vi "ParseBounceData.vi"(5 "Data_In":string="b'OK\\n\\r'\r\nDMA Length: 43008\r\nTx_1 Rx_1: {'Frequency': 'Passed', 'Power': 'Passed'}\r\nMax Value: -5.066 dBFS at -6.226 MHz\r\nTx_2 Rx_1: {'Frequency': 'Passed', 'Power': 'Passed'}\r\nMax Value: -6.924 dBFS at -6.226 MHz\r\nTx_1 Rx_2: {'Frequency': 'Passed', 'Power': 'Passed'}\r\nMax Value: -6.565 dBFS at -6.152 MHz\r\nTx_3 Rx_1: {'Frequency': 'Passed', 'Power': 'Passed'}\r\nMax Value: -6.967 dBFS at -6.226 MHz\r\nTx_2 Rx_2: {'Frequency': 'Passed', 'Power': 'Passed'}\r\nMax Value: -6.388 dBFS at -6.226 MHz\r\nTx_4 Rx_1: {'Frequency': 'Passed', 'Power': 'Passed'}\r\nMax Value: -6.945 dBFS at -6.226 MHz\r\nTx_3 Rx_2: {'Frequency': 'Passed', 'Power': 'Passed'}\r\nMax Value: -6.080 dBFS at -6.152 MHz\r\nTx_2 Rx_3: {'Frequency': 'Passed', 'Power': 'Passed'}\r\nMax Value: -5.226 dBFS at -6.152 MHz\r\nTx_4 Rx_2: {'Frequency': 'Passed', 'Power': 'Passed'}\r\nMax Value: -6.517 dBFS at -6.226 MHz\r\nTx_3 Rx_3: {'Frequency': 'Passed', 'Power': 'Passed'}\r\nMax Value: -5.453 dBFS at -6.226 MHz\r\nTx_5 Rx_2: {'Frequency': 'Passed', 'Power': 'Passed'}\r\nMax Value: -6.717 dBFS at -6.226 MHz\r\nTx_4 Rx_3: {'Frequency': 'Passed', 'Power': 'Passed'}\r\nMax Value: -5.646 dBFS at -6.226 MHz\r\nTx_3 Rx_4: {'Frequency': 'Passed', 'Power': 'Passed'}\r\nMax Value: -5.349 dBFS at -6.152 MHz\r\nTx_5 Rx_3: {'Frequency': 'Passed', 'Power': 'Passed'}\r\nMax Value: -5.643 dBFS at -6.226 MHz\r\nTx_4 Rx_4: {'Frequency': 'Passed', 'Power': 'Passed'}\r\nMax Value: -5.707 dBFS at -6.226 MHz\r\nTx_6 Rx_3: {'Frequency': 'Passed', 'Power': 'Passed'}\r\nMax Value: -5.844 dBFS at -6.226 MHz\r\nTx_5 Rx_4: {'Frequency': 'Passed', 'Power': 'Passed'}\r\nMax Value: -5.505 dBFS at -6.226 MHz\r\nTx_7 Rx_3: {'Frequency': 'Passed', 'Power': 'Passed'}\r\nMax Value: -5.223 dBFS at -6.152 MHz\r\nTx_6 Rx_4: {'Frequency': 'Passed', 'Power': 'Passed'}\r\nMax Value: -5.202 dBFS at -6.226 MHz\r\nTx_5 Rx_5: {'Frequency': 'Passed', 'Power': 'Passed'}\r\nMax Value: -5.983 dBFS at -6.226 MHz\r\nTx_7 Rx_4: {'Frequency': 'Passed', 'Power': 'Passed'}\r\nMax Value: -5.318 dBFS at -6.226 MHz\r\nTx_6 Rx_5: {'Frequency': 'Passed', 'Power': 'Passed'}\r\nMax Value: -5.734 dBFS at -6.226 MHz\r\nTx_8 Rx_4: {'Frequency': 'Passed', 'Power': 'Passed'}\r\nMax Value: -5.205 dBFS at -6.226 MHz\r\nTx_7 Rx_5: {'Frequency': 'Passed', 'Power': 'Passed'}\r\nMax Value: -5.248 dBFS at -6.226 MHz\r\nTx_6 Rx_6: {'Frequency': 'Passed', 'Power': 'Passed'}\r\nMax Value: -5.428 dBFS at -6.226 MHz\r\nTx_8 Rx_5: {'Frequency': 'Passed', 'Power': 'Passed'}\r\nMax Value: -5.738 dBFS at -6.226 MHz\r\nTx_7 Rx_6: {'Frequency': 'Passed', 'Power': 'Passed'}\r\nMax Value: -5.289 dBFS at -6.226 MHz\r\nTx_9 Rx_5: {'Frequency': 'Passed', 'Power': 'Passed'}\r\nMax Value: -6.211 dBFS at -6.226 MHz\r\nTx_8 Rx_6: {'Frequency': 'Passed', 'Power': 'Passed'}\r\nMax Value: -5.201 dBFS at -6.226 MHz\r\nTx_10 Rx_5: {'Frequency': 'Passed', 'Power': 'Passed'}\r\nMax Value: -6.328 dBFS at -6.226 MHz\r\nTx_9 Rx_6: {'Frequency': 'Passed', 'Power': 'Passed'}\r\nMax Value: -6.355 dBFS at -6.226 MHz\r\nTx_8 Rx_7: {'Frequency': 'Passed', 'Power': 'Passed'}\r\nMax Value: -5.296 dBFS at -6.226 MHz\r\nTx_10 Rx_6: {'Frequency': 'Passed', 'Power': 'Passed'}\r\nMax Value: -6.349 dBFS at -6.226 MHz\r\nTx_9 Rx_7: {'Frequency': 'Passed', 'Power': 'Passed'}\r\nMax Value: -6.183 dBFS at -6.226 MHz\r\nTx_11 Rx_6: {'Frequency': 'Passed', 'Power': 'Passed'}\r\nMax Value: -6.896 dBFS at -6.226 MHz\r\nTx_10 Rx_7: {'Frequency': 'Passed', 'Power': 'Passed'}\r\nMax Value: -6.724 dBFS at -6.226 MHz\r\nTx_9 Rx_8: {'Frequency': 'Passed', 'Power': 'Passed'}\r\nMax Value: -6.414 dBFS at -6.226 MHz\r\nTx_11 Rx_7: {'Frequency': 'Passed', 'Power': 'Passed'}\r\nMax Value: -6.283 dBFS at -6.226 MHz\r\nTx_10 Rx_8: {'Frequency': 'Passed', 'Power': 'Passed'}\r\nMax Value: -6.328 dBFS at -6.226 MHz\r\nTx_12 Rx_7: {'Frequency': 'Passed', 'Power': 'Passed'}\r\nMax Value: -5.939 dBFS at -6.226 MHz\r\nTx_11 Rx_8: {'Frequency': 'Passed', 'Power': 'Passed'}\r\nMax Value: -6.370 dBFS at -6.226 MHz\r\nTx_12 Rx_8: {'Frequency': 'Passed', 'Power': 'Passed'}\r\nMax Value: -6.672 dBFS at -6.226 MHz\r\n", 11 "error in":errorcluster) -> (2 "P/F_power":bool, 3 "Passed?(T)":bool, 6 "Data_Out":string[][](array[string]), 15 "error out":errorcluster)   [LabVIEW 2018]
panel:
  out "P/F_freq":bool[](array[boolean])
  out "Array 3":string[](array[string])
  out "Array 2":string[](array[string])
  out "mhz":string[](array[string])
  out "dbfs":string[](array[string])
  out "rx":string[](array[string])
  out "tx":string[](array[string])
  out "Formatted_ary":string[][](array[string])
  out "size_match?(t)":bool
  out "Data_index":i32[](array[numeric])
  out "Tx_index":i32[](array[numeric])
  out "spreadsheet string":string
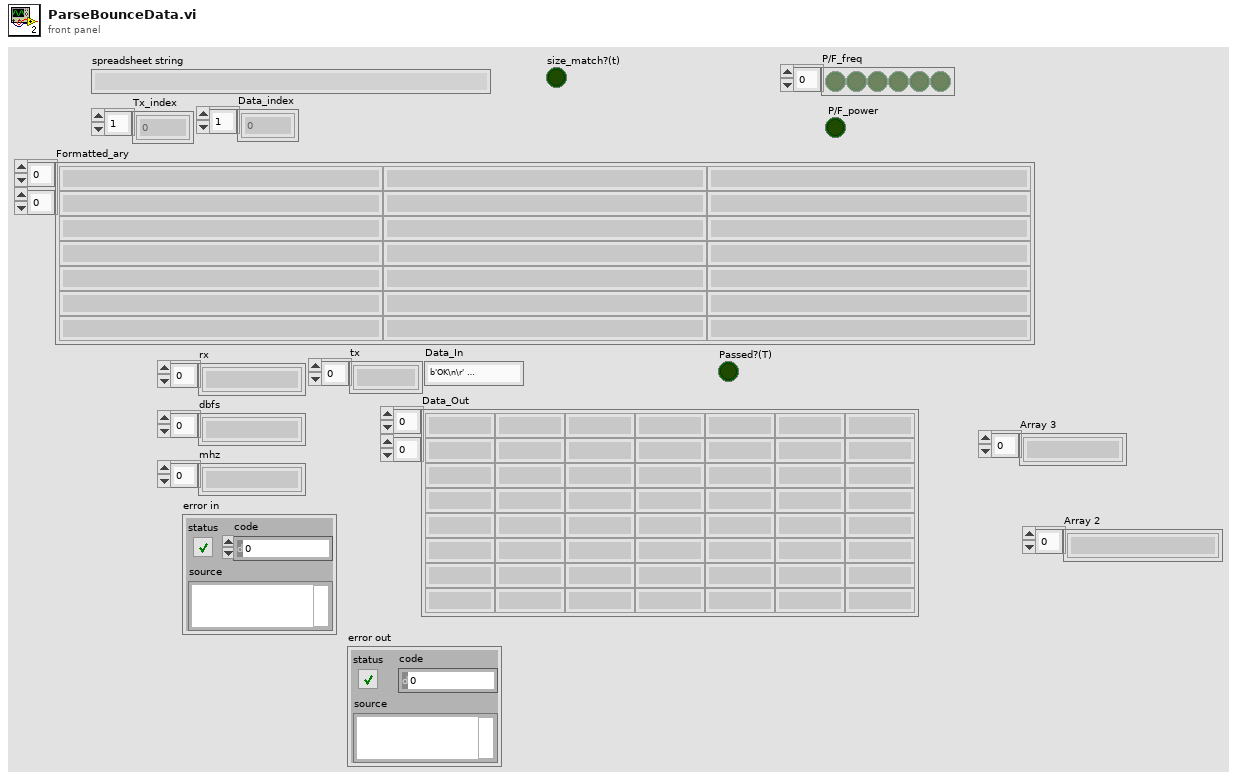
[diagram p1: front panel]
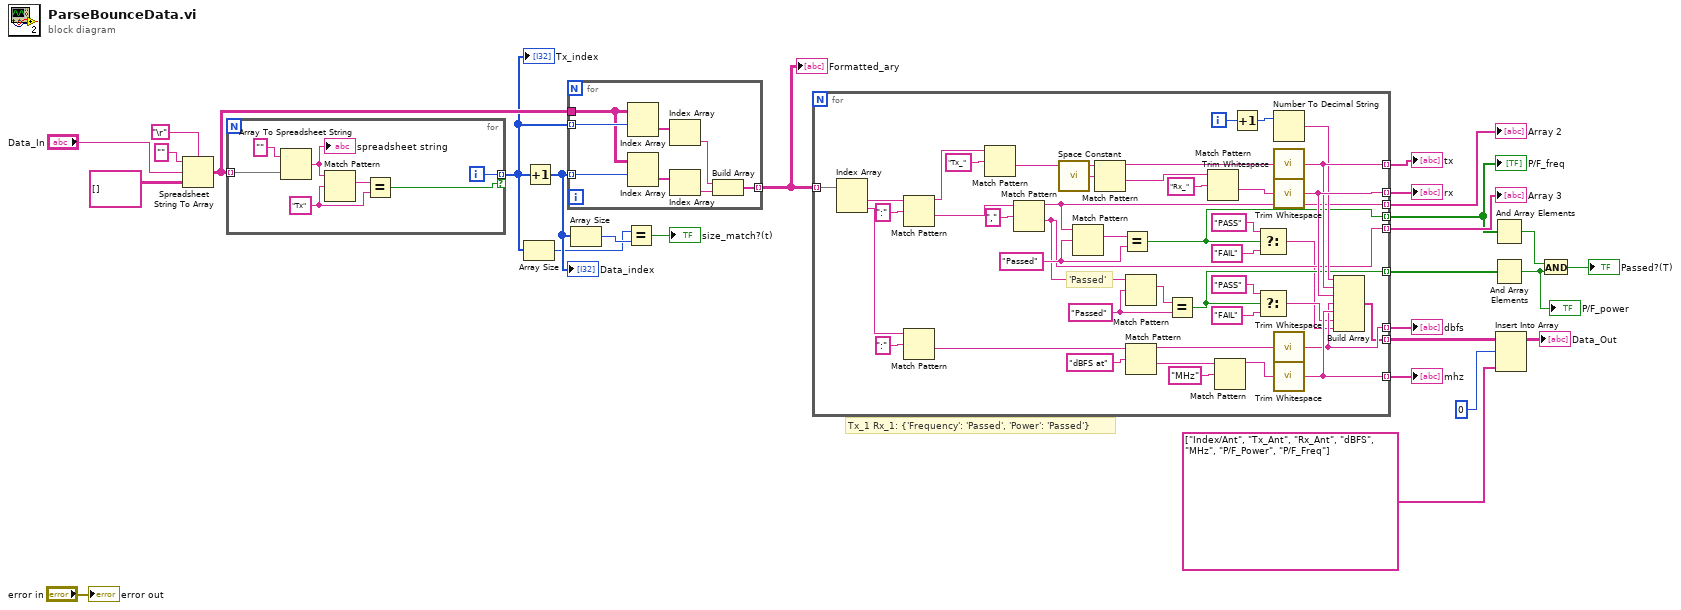
[diagram p0: block diagram]
diagram:
  # "Tx_1 Rx_1: {'Frequency': 'Passed', 'Power': 'Passed'}"
  n1 = Spreadsheet String To Array(delimiter (Tab)="\r", format string="", spreadsheet string="Data_In", array type (2D Dbl)=string[][] []) -> (array=w23:string[][])
  n2 = for {
    tunnel: w23 -> [w34] mode=indexing
    tunnel: [w29] -> w21 mode=indexing if=w28
    i -> [w29]
    w30 = "Tx" ("regular expression")
    n3 = Array To Spreadsheet String(array=w34, 3:"" ("format string")) -> (spreadsheet string=w32:string)  [unwired: 1 in]
    "spreadsheet string" <- w32
    n4 = Match Pattern(string=w32, regular expression=w30) -> (match substring=w31:string)  [unwired: 1 in, 3 out]
    n5 = Equal?(x=w31, y=w30) -> (x = y?=w28:bool)
  }
  "Tx_index" <- w21
  n6 = Array Size(array=w21) -> (size(s)=w19:i32)
  n7 = Increment(x=w21) -> (x+1=w22:i32[])
  "Data_index" <- w22
  n8 = for {
    tunnel: w23 -> [w39]
    tunnel: w22 -> [w42] mode=indexing
    tunnel: w21 -> [w40] mode=indexing
    tunnel: [w35] -> w17 mode=indexing
    n9 = Index Array(array=w39, index (row)=w40) -> (element=w38:string[])  [unwired: 1 in]
    n10 = Index Array(array=w39, index (row)=w42) -> (element=w41:string[])  [unwired: 1 in]
    n11 = Index Array(array=w38) -> (element=w37:string)  [unwired: 1 in]
    n12 = Index Array(array=w41) -> (element=w36:string)  [unwired: 1 in]
    n13 = Build Array(w37, w36) -> (w35:string[])
  }
  "Formatted_ary" <- w17
  n14 = Array Size(array=w22) -> (size(s)=w20:i32)
  n15 = Equal?(x=w19, y=w20) -> (x = y?=→"size_match?(t)":bool)
  n16 = for {
    tunnel: w17 -> [w85] mode=indexing
    tunnel: [w63] -> w16 mode=indexing
    tunnel: [w64] -> w15 mode=indexing
    tunnel: [w65] -> w14 mode=indexing
    tunnel: [w66] -> w13 mode=indexing
    tunnel: [w62] -> w12 mode=indexing
    tunnel: [w56] -> w8 mode=indexing
    tunnel: [w51] -> w7 mode=indexing
    tunnel: [w50] -> w6 mode=indexing
    tunnel: [w45] -> w5 mode=indexing
    i -> [w60]
    w53 = "Passed"
    w54 = "Passed"
    # "'Passed'"
    n17 = Index Array(array=w85) -> (element #1=w77:string, element #2=w73:string)  [unwired: 2 in]
    n18 = Match Pattern(string=w77, regular expression=":") -> (before substring=w81:string, after substring=w58:string)  [unwired: 1 in, 2 out]
    n19 = Match Pattern(string=w73, regular expression=":") -> (after substring=w72:string)  [unwired: 1 in, 3 out]
    n20 = Match Pattern(string=w81, regular expression="Tx_") -> (after substring=w80:string)  [unwired: 1 in, 3 out]
    n21 = Match Pattern(string=w58, regular expression=",") -> (before substring=w56:string, after substring=w51:string)  [unwired: 1 in, 2 out]
    n22 = call <vilib>:"Space Constant.vi"() -> ("String"=w79:string)
    n23 = Match Pattern(string=w56, regular expression=w54) -> (match substring=w55:string)  [unwired: 1 in, 3 out]
    n24 = Match Pattern(string=w80, regular expression=w79) -> (before substring=w78:string, after substring=w76:string)  [unwired: 1 in, 2 out]
    n25 = Equal?(x=w55, y=w54) -> (x = y?=w50:bool)
    n26 = Match Pattern(string=w51, regular expression=w53) -> (match substring=w52:string)  [unwired: 1 in, 3 out]
    n27 = Match Pattern(string=w72, regular expression="dBFS at") -> (before substring=w70:string, after substring=w69:string)  [unwired: 1 in, 2 out]
    n28 = Equal?(x=w52, y=w53) -> (x = y?=w45:bool)
    n29 = Match Pattern(string=w76, regular expression="Rx_") -> (after substring=w75:string)  [unwired: 1 in, 3 out]
    n30 = Match Pattern(string=w69, regular expression="MHz") -> (before substring=w67:string)  [unwired: 1 in, 3 out]
    n31 = Increment(x=w60) -> (x+1=w59:i32)
    n32 = Select(t="PASS", s=w50, f="FAIL") -> (s? t:f=w43:string)
    n33 = Select(t="PASS", s=w45, f="FAIL") -> (s? t:f=w44:string)
    n34 = Number To Decimal String(number=w59) -> (decimal integer string=w61:string)  [unwired: 1 in]
    n35 = call <vilib>:"Trim Whitespace.vi"("string"=w78) -> ("trimmed string"=w63:string)  [unwired: 1 in]
    n36 = call <vilib>:"Trim Whitespace.vi"("string"=w75) -> ("trimmed string"=w64:string)  [unwired: 1 in]
    n37 = call <vilib>:"Trim Whitespace.vi"("string"=w70) -> ("trimmed string"=w65:string)  [unwired: 1 in]
    n38 = call <vilib>:"Trim Whitespace.vi"("string"=w67) -> ("trimmed string"=w66:string)  [unwired: 1 in]
    n39 = Build Array(w61, w63, w64, w65, w66, w44, w43) -> (w62:string[])
  }
  "tx" <- w16
  "rx" <- w15
  "dbfs" <- w14
  "mhz" <- w13
  "Array 2" <- w8
  "Array 3" <- w7
  "P/F_freq" <- w6
  n40 = And Array Elements(Boolean array=w6) -> (logical AND=w4:bool)
  n41 = And Array Elements(Boolean array=w5) -> (logical AND=w1:bool)
  "P/F_power" <- w1
  n42 = Insert Into Array(array=w12, index (row)=0, new element=string[] ["Index/Ant", "Tx_Ant", "Rx_Ant", "dBFS", "MHz", "P/F_Power", "P/F_Freq"] ("new element/subarray")) -> (→"Data_Out":string[][])  [unwired: 1 in]
  n43 = And(x=w4, y=w1) -> (x .and. y?=→"Passed?(T)":bool)
  "error out" <- "error in"
